vi "CRYAPI Pic CheckSplitterSubPanelOver.vi"   [LabVIEW 2013]
uses:
  CRYMain Sub Window Global.vi
types:
  T1 = cluster{"nID":i32[], "Spliter":cluster{"nType":i32, "nTypeP":i32, "pVI":refnum<vi>, "pSpliter":refnum<vi>, "pSPL":refnum<vi>, "pVIL":refnum<vi>, "pSPR":refnum<vi>, "pVIR":refnum<vi>, "nIDTL":i32, "nIDL":i32, "nIDTR":i32, "nIDR":i32, "nID":i32, "nIDParent":i32, "nData":i32, "sData":string}[]}
  T2 = cluster{"nType":i32, "nTypeP":i32, "pVI":refnum<vi>, "pSpliter":refnum<vi>, "pSPL":refnum<vi>, "pVIL":refnum<vi>, "pSPR":refnum<vi>, "pVIR":refnum<vi>, "nIDTL":i32, "nIDL":i32, "nIDTR":i32, "nIDR":i32, "nID":i32, "nIDParent":i32, "nData":i32, "sData":string}[]
  T3 = typedef "LVBoundsTypeDef.ctl" = cluster{"Width":u32, "Height":u32}
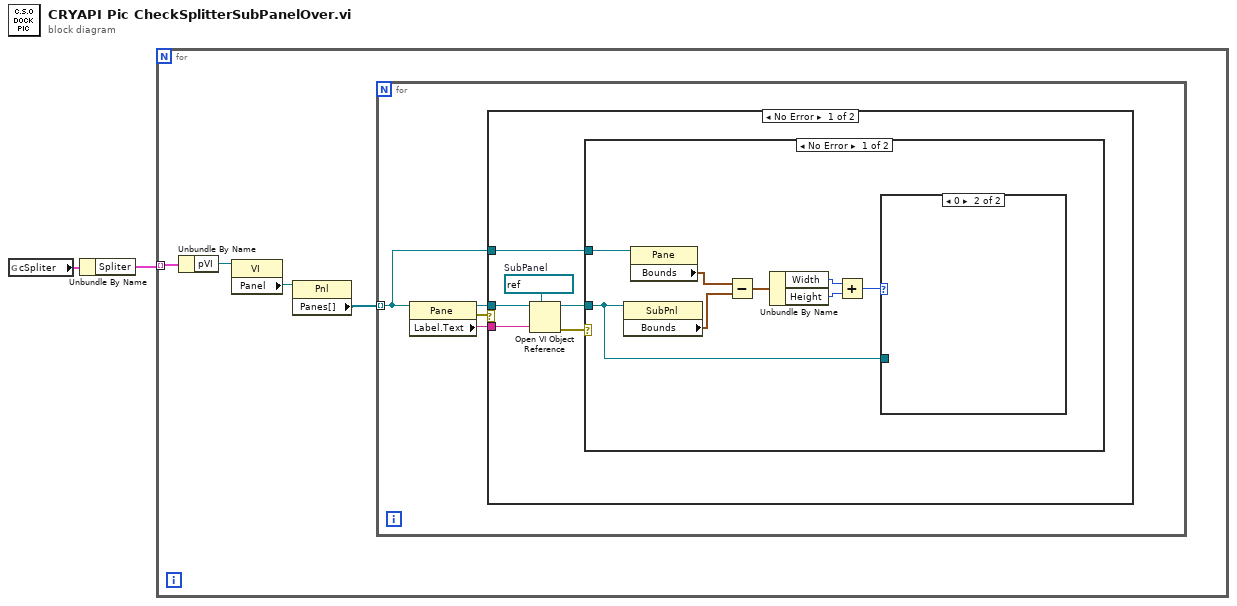
[diagram p0: block diagram]
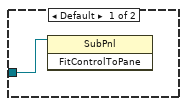
[diagram p2: hidden frame]
diagram:
  n1 = global read "CRYMain Sub Window Global.vi" "cSpliter"() -> (w2:T1)
  n2 = Unbundle By Name(w2) -> ("Spliter"=w1:T2)
  n3 = for {
    tunnel: w1 -> [w4] mode=indexing
    n4 = Unbundle By Name(w4) -> ("pVI"=w3:refnum<vi>)
    n5 = property class="VI"(reference=w3) -> ("Panel"=w6:refnum<vi>)  [unwired: 1 in, 2 out]
    n6 = property class="Pnl"(reference=w6) -> ("Panes[]"=w5:refnum<vi>[])  [unwired: 1 in, 2 out]
    n7 = for {
      tunnel: w5 -> [w7] mode=indexing
      n8 = property class="Pane"(reference=w7) -> (reference out=w9:refnum<vi>, error out=w8:errorcluster, "Label.Text"=w10:string)  [unwired: 1 in]
      n9 = case shown="No Error" w8 {
        tunnel: w10 -> [w15 _]
        tunnel: w9 -> [w14 _]
        tunnel: w7 -> [w11 _]
        frame No Error {
          w16 = refnum<vi> refnum  # SubPanel
          n10 = Open VI Object Reference(7:w16, 10:w15, 11:w14) -> (0:w13:errorcluster, 3:w12:refnum<vi>)  [unwired: 1 in]
          n11 = case shown="No Error" w13 {
            tunnel: w12 -> [w17 _]
            tunnel: w11 -> [w24 _]
            frame No Error {
              n12 = property class="SubPnl"(reference=w17) -> ("Bounds"=w22:T3)  [unwired: 1 in, 2 out]
              n13 = property class="Pane"(reference=w24) -> ("Bounds"=w23:T3)  [unwired: 1 in, 2 out]
              n14 = Subtract(x=w23, y=w22) -> (x-y=w21:T3)
              n15 = Unbundle By Name(w21) -> ("Width"=w20:u32, "Height"=w19:u32)
              n16 = Add(x=w20, y=w19) -> (x+y=w18:u32)
              n17 = case shown="0" w18 {
                tunnel: w17 -> [w25 _]
                frame Default {
                  n18 = invoke class="SubPnl" method="FitControlToPane"(reference=w25) -> ()  [unwired: 2 in, 3 out]
                }
                frame 0 {
                }
              }
            }
            frame Error {
            }
          }
        }
        frame Error {
        }
      }
    }
  }
